vi "TIRF_SetLEDStrings.vi"(8 "error in (no error)":errorcluster, 9 "Value":string="No Pulse", 10 "LED Values":T1(array[cluster]), 11 "Select Filter:":refnum<vi>) -> (0 "error out":errorcluster)   [LabVIEW 2010]
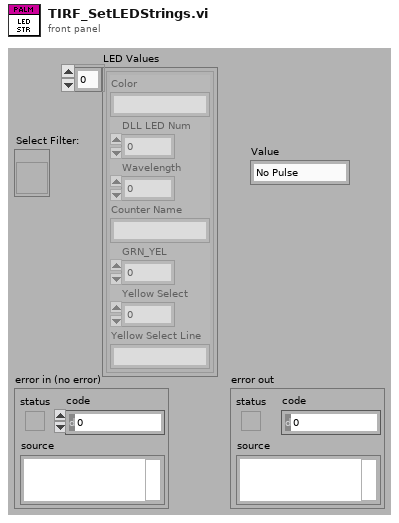
[diagram p1: front panel]
types:
  T1 = cluster{"Color":string, "DLL LED Num":i32, "Wavelength":i32, "Counter Name":string, "GRN_YEL":i32, "Yellow Select":i32, "Yellow Select Line":string}[]
  T2 = cluster{"format string":string, "format string":string}
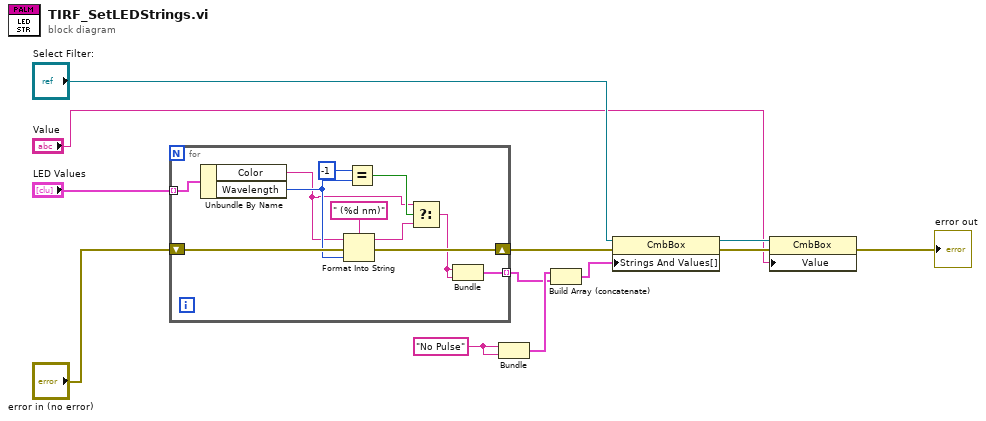
[diagram p0: block diagram]
diagram:
  w3 = "No Pulse" ("format string")
  n1 = for {
    tunnel: "LED Values" -> [w23] mode=indexing
    shift-right: [w21] -> w11
    shift-left: "error in (no error)" -> [w22]
    tunnel: [w19] -> w1 mode=indexing
    n2 = Unbundle By Name(w23) -> ("Color"=w14:string, "Wavelength"=w18:i32)
    n3 = Format Into String(format string=" (%d nm)", initial string=w14, error in=w22, w18) -> (resulting string=w15:string, error out=w21:errorcluster)
    n4 = Equal?(x=-1, y=w18) -> (x = y?=w16:bool)
    n5 = Select(t=w14, s=w16, f=w15) -> (s? t:f=w13:string)
    n6 = Bundle("Color"=w13, "Color"=w13) -> (w19:cluster{"Color":string, "Color":string})  [unwired: 1 in]
  }
  n7 = Bundle("format string"=w3, "format string"=w3) -> (w2:T2)  [unwired: 1 in]
  n8 = Build Array (concatenate)(w2, w1) -> (w4:cluster{"Color":string, "Color":string}[])
  n9 = property on="Property Node" class="CmbBox"(reference="Select Filter:", error in=w11, "Strings And Values[]"=w4) -> (reference out=w8:refnum<vi>, error out=w9:errorcluster)
  n10 = property on="Property Node" class="CmbBox"(reference=w8, error in=w9, "Value"="Value") -> (error out=→"error out":errorcluster)  [unwired: 1 out]
